vi "OpenIOMonitor.vi"   [LabVIEW 2021]
uses:
  <vilib>/registry/registry.llb/Registry SAM.ctl
  <vilib>/registry/registry.llb/Registry RtKey.ctl
  <vilib>/registry/registry.llb/Read Registry Value Simple STR.vi
types:
  T1 = typedef "Registry SAM.ctl" = enum32{"KEY_QUERY_VALUE", "KEY_SET_VALUE", "KEY_CREATE_SUB_KEY", "KEY_ENUMERATE_SUB_KEYS", "KEY_NOTIFY", "KEY_CREATE_LINK", "KEY_READ", "KEY_WRITE", "KEY_ALL_ACCESS", "KEY_READ | KEY_WRITE"}
  T2 = typedef "Registry RtKey.ctl" = enum32{"HKEY_CLASSES_ROOT", "HKEY_CURRENT_USER", "HKEY_LOCAL_MACHINE", "HKEY_USERS", "HKEY_PERFORMANCE_DATA", "HKEY_CURRENT_CONFIG", "HKEY_DYN_DATA"}
  T3 = typedef "Registry refnum.ctl" = refnum<k1>
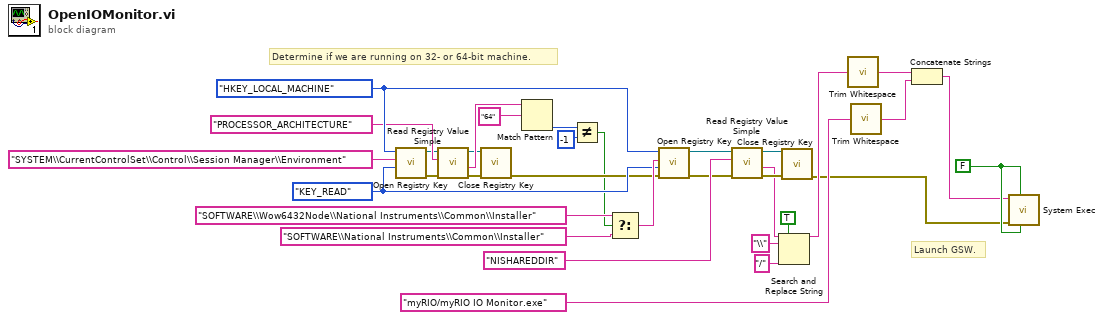
[diagram p0: block diagram]
diagram:
  w7 = FALSE ("wait until completion? (T)")
  w26 = Registry_SAM."KEY_READ" ("security access mask (KEY_READ | KEY_WRITE)")
  w25 = Registry_RtKey."HKEY_LOCAL_MACHINE" ("root key (HKEY_LOCAL_MACHINE)")
  # "Determine if we are running on 32- or 64-bit machine."
  # "Launch GSW."
  n1 = call <vilib>:"Open Registry Key.vi"("security access mask (KEY_READ | KEY_WRITE)"=w26, "subkey"="SYSTEM\\CurrentControlSet\\Control\\Session Manager\\Environment", "root key (HKEY_LOCAL_MACHINE)"=w25) -> ("error out"=w11:errorcluster, "refnum out"=w10:T3)  [unwired: 1 in, 6 out]
  n2 = call-poly <vilib>:"Read Registry Value Simple.vi"("error in (no error)"=w11, "value"="PROCESSOR_ARCHITECTURE", "refnum"=w10) -> ("error out"=w14:errorcluster, "String/Binary data"=w15:string, "refnum out"=w13:T3)  [unwired: 1 in, 3 out]
  n3 = call <vilib>:"Close Registry Key.vi"("error in (no error)"=w14, "refnum"=w13) -> ("error out"=w22:errorcluster)  [unwired: 5 out]
  n4 = Match Pattern(string=w15, regular expression="64") -> (offset past match=w17:i32)  [unwired: 4 out]
  n5 = Not Equal?(x=w17, y=-1) -> (x != y?=w19:bool)
  n6 = Select(t="SOFTWARE\\Wow6432Node\\National Instruments\\Common\\Installer" ("string"), s=w19, f="SOFTWARE\\National Instruments\\Common\\Installer" ("string")) -> (s? t:f=w27:string)
  n7 = call <vilib>:"Open Registry Key.vi"("error in (no error)"=w22, "security access mask (KEY_READ | KEY_WRITE)"=w26, "subkey"=w27, "root key (HKEY_LOCAL_MACHINE)"=w25) -> ("error out"=w24:errorcluster, "refnum out"=w23:T3)  [unwired: 6 in]
  n8 = call-poly <vilib>:"Read Registry Value Simple.vi"("error in (no error)"=w24, "value"="NISHAREDDIR", "refnum"=w23) -> ("error out"=w30:errorcluster, "String/Binary data"=w8:string, "refnum out"=w29:T3)  [unwired: 3 in, 1 out]
  n9 = Search and Replace String(replace all?=TRUE ("replace all? (F)"), input string=w8, search string="\\", replace string="/" ("replace string (\"\")")) -> (result string=w5:string)  [unwired: 4 in, 3 out]
  n10 = call <vilib>:"Close Registry Key.vi"("error in (no error)"=w30, "refnum"=w29) -> ("error out"=w2:errorcluster)  [unwired: 5 out]
  n11 = call <vilib>:"Trim Whitespace.vi"("string"=w5) -> ("trimmed string"=w6:string)  [unwired: 1 in]
  n12 = call <vilib>:"Trim Whitespace.vi"("string"="myRIO/myRIO IO Monitor.exe" ("input 2")) -> ("trimmed string"=w4:string)  [unwired: 1 in]
  n13 = Concatenate Strings(w6, w4) -> (w1:string)
  n14 = call <vilib>:"System Exec.vi"("run minimized? (F)"=w7, "wait until completion? (T)"=w7, "error in (no error)"=w2, "command line"=w1) -> ()  [unwired: 4 in, 4 out]
